vi "SUB_Shutdown_Telnet.vi"() -> ()   [LabVIEW 2011]
panel:
  out "Telnet Ok ?":bool
  out "Found":bool
  out "msg out":string
  # "Step1:¥ýtelnet log in\nStep2:get root authority\nStep3:ShutDown"
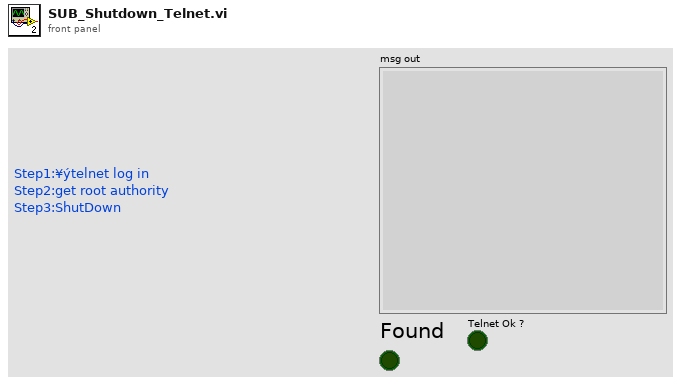
[diagram p1: front panel]
types:
  T1 = typedef "Telnet Session.ctl" = refnum<k1>
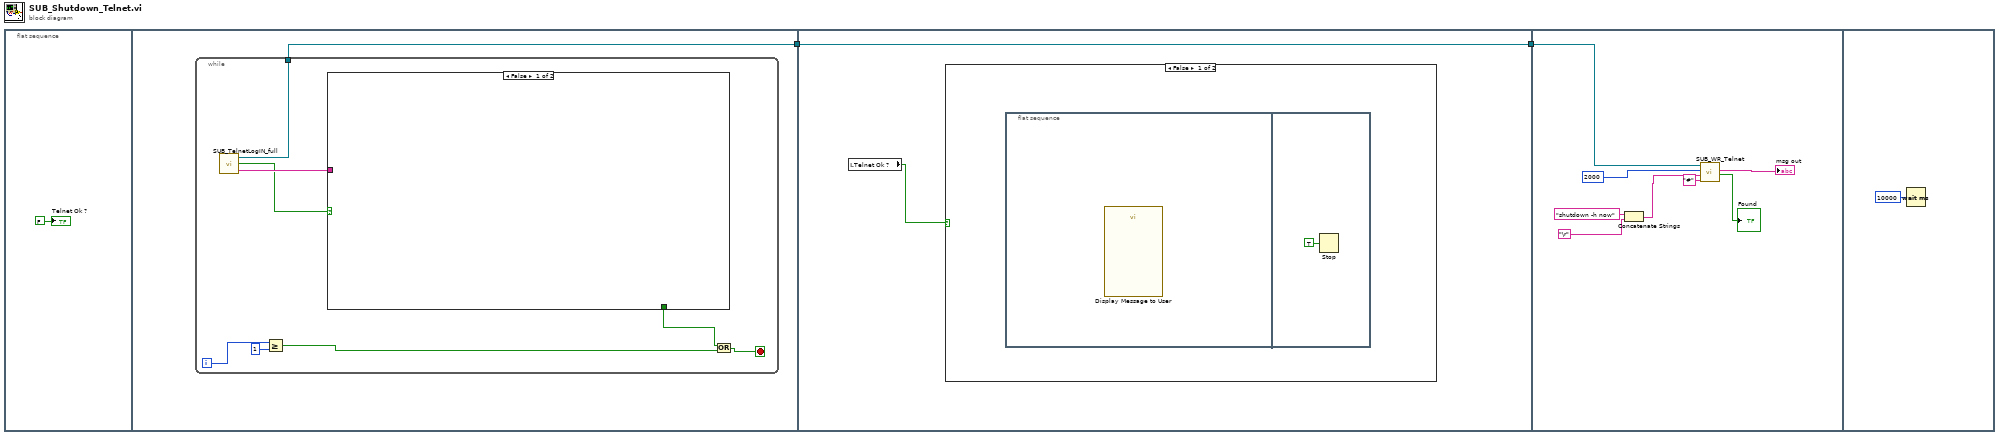
[diagram p0: block diagram]
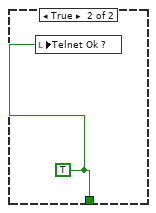
[diagram p2: hidden frame]
diagram:
  n1 = flat-sequence {
    tunnel: [w4] -> w2
    tunnel: w2 -> [w15]
    tunnel: [w15] -> w1
    tunnel: w1 -> [w24]
    frame #0 {
      "Telnet Ok ?" <- FALSE
    }
    frame #1 {
      n2 = while {
        tunnel: [w11] -> w4
        i -> [w7]
        stop <- w9 stop-if-true
        n3 = call "SUB_TelnetLogIN_full.vi"() -> ("telnet connection"=w11:T1, "Pass ?"=w10:bool, "data out"=w12:string)  [unwired: 2 in]
        n4 = Greater Or Equal?(x=w7, y=1) -> (x >= y?=w5:bool)
        n5 = case shown="False" w10 {
          tunnel: w12 -> [_ _]
          tunnel: [_ w13] -> w8
          frame False {
          }
          frame True {
            w13 = TRUE
            n6 = local write "Telnet Ok ?"(w13) -> ()
          }
        }
        n7 = Or(x=w8, y=w5) -> (x .or. y?=w9:bool)
      }
    }
    frame #2 {
      n8 = local read "Telnet Ok ?"() -> (w14:bool)
      n9 = case shown="False" w14 {
        frame False {
          n10 = flat-sequence {
            frame #0 {
              n11 = call "Display Message to User"() -> ()  [unwired: 10 in, 2 out]
            }
            frame #1 {
              n12 = Stop(stop? (T)=TRUE) -> ()
            }
          }
        }
        frame True {
        }
      }
    }
    frame #3 {
      n13 = Concatenate Strings("shutdown -h now" ("string"), "\r") -> (w20:string)
      n14 = call "SUB_WR_Telnet.vi"("Find this String"="#", "data in"=w20, "timeout ms"=2000, "telnet connection"=w24) -> ("Found"=→"Found":bool, "msg out"=→"msg out":string)  [unwired: 1 in, 1 out]
    }
    frame #4 {
      n15 = Wait (ms)(milliseconds to wait=u32 10000) -> ()  [unwired: 1 out]
    }
  }
